vi "Test Image Display.vi"(10 "Point":cluster{"X":i32, "Y":i32}, 11 "Image In":T1(plugin-control)) -> (3 "Image":T1)   [LabVIEW 2013]
uses:
  <vilib>/vision/Image Controls.llb/IMAQ Image.ctl
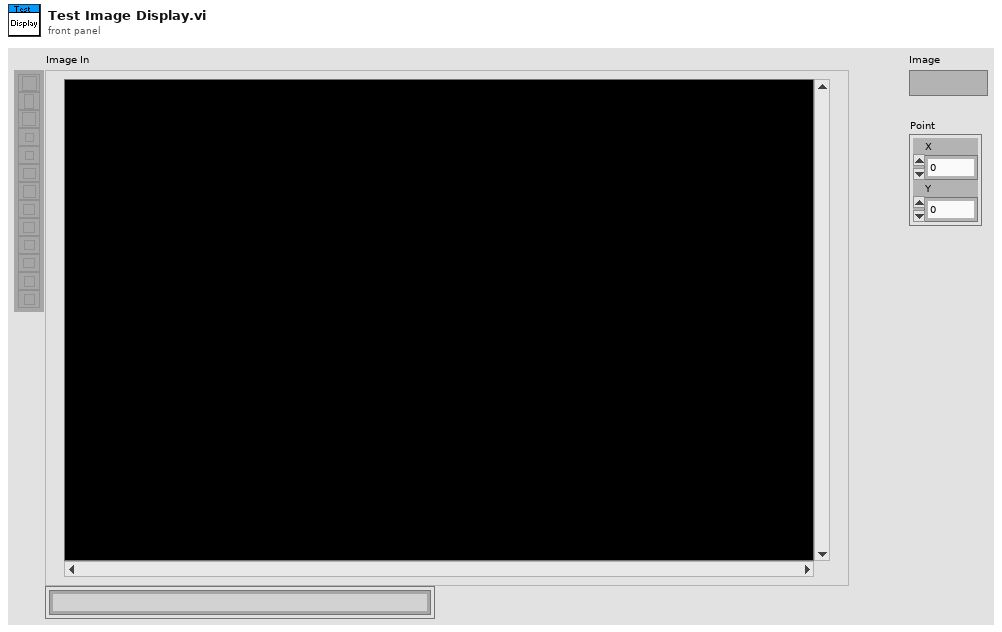
[diagram p1: front panel]
types:
  T1 = typedef "IMAQ Image.ctl" = refnum<image>
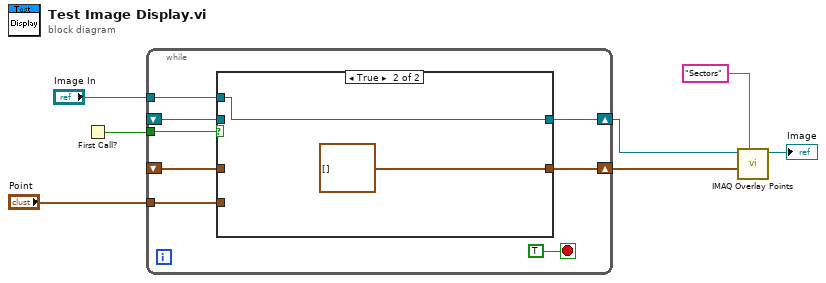
[diagram p0: block diagram]
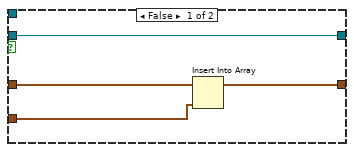
[diagram p2: hidden frame]
diagram:
  n1 = First Call?() -> (First Call?: T/F=w4:bool)
  n2 = while {
    tunnel: "Point" -> [w15]
    shift-right: [w13] -> w5
    shift-left: _ -> [w14]
    tunnel: w4 -> [w11]
    tunnel: "Image In" -> [w9]
    shift-right: [w10] -> w2
    shift-left: _ -> [w8]
    stop <- TRUE stop-if-true
    n3 = case shown="True" w11 {
      tunnel: w15 -> [w17 _]
      tunnel: w14 -> [w18 _]
      tunnel: [w16 cluster{"X":i32, "Y":i32}[] [] ("Array of Points")] -> w13
      tunnel: [w19 w20] -> w10
      tunnel: w9 -> [_ w20]
      tunnel: w8 -> [w19 _]
      frame False {
        n4 = Insert Into Array(array=w18, new element=w17) -> (w16:cluster{"X":i32, "Y":i32}[])  [unwired: 1 in]
      }
      frame True {
      }
    }
  }
  n5 = call "IMAQ Overlay Points"("Group"="Sectors", "Array of Points"=w5, "Image"=w2) -> ("Image Out"=→"Image":T1)  [unwired: 7 in, 1 out]
